vi "PH_Beckhoff_PP_PU.get Igni Tagname.vi"(1 "Igni Tag":T2, 2 "PU":T1) -> (0 "Igni Tagname":string)   [LabVIEW 2014, in "PH_Beckhoff_PP_PU.lvlib"]
doc: "This VI concatenates a Tagname out of strict type def enum controls. It keeps also the information whether the Tag is existing (if not, N/A is given out as name)."
uses:
  PH_Beckhoff_PP_PU.lvlib
  PH_Beckhoff_PP_PU.Igni Tags.ctl
  PH_PP_Common/PH_PP_Common.PUs.ctl
  PH_PP_Common/PH_PP_Common.Devices.ctl
  PH_Common/Names/PH_Names.Subsystems.ctl
  PH_Common/Names/PH_Names.Communication Type.ctl
  PH_Common/PH_Common.lvlib
  PH_PP_Common/PH_PP_Common.lvlib
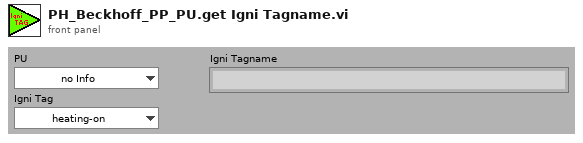
[diagram p1: front panel]
types:
  T1 = typedef "PH_PP_Common.lvlib/PH_PP_Common.PUs.ctl" = enum16{"no Info", "PA-19mm-1", "PA-19mm-2", "PA-45mm-PILC", "PA-45mm-MAIN", "MA-PU-1", "MA-PU-2", "MA-PU-3", "MA-PU-4", "MA-PU-5", "MA-PU-6", "MA-FR", "MA-PILC", "PA-45mm-DP"}
  T2 = typedef "PH_Beckhoff_PP_PU.lvlib/PH_Beckhoff_PP_PU.Igni Tags.ctl" = enum16{"heating-on", "water-on", "Device-on", "Status"}
  T3 = typedef "PH_Common.lvlib/PH_Names.Subsystems.ctl" = enum16{"no Info", "fs-FE", "ns-FE", "PA", "MA", "MAS", "COS", "Exp-LB", "Exp-LL", "PP", "PILS"}
  T4 = typedef "PH_PP_Common.lvlib/PH_PP_Common.Devices.ctl" = enum16{"no Info", "Igni", "RR", "DumpRoss", "PSU", "Trigger", "HV-Meas", "Rods", "Chiller", "Conductivity", "Mercury"}
  T5 = typedef "PH_Common.lvlib/PH_Names.Communication Type.ctl" = enum16{"no Info", "SE", "SA", "AE", "AA", "DE", "DA", "DIM"}
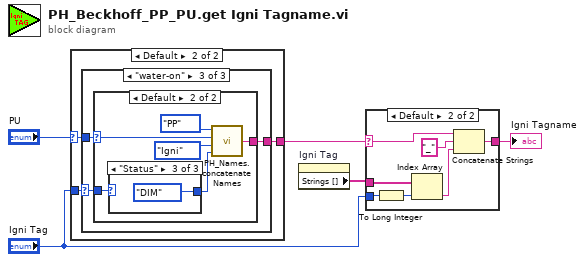
[diagram p0: block diagram]
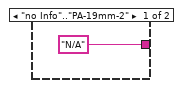
[diagram p2: hidden frame]
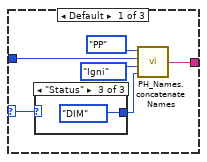
[diagram p3: hidden frame]
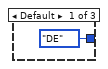
[diagram p4: hidden frame]
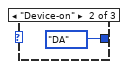
[diagram p5: hidden frame]
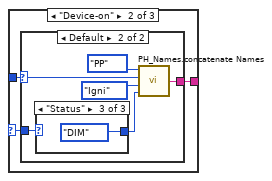
[diagram p6: hidden frame]
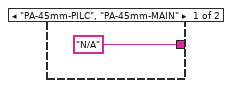
[diagram p7: hidden frame]
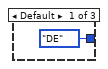
[diagram p8: hidden frame]
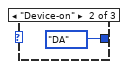
[diagram p9: hidden frame]
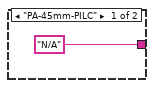
[diagram p10: hidden frame]
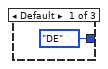
[diagram p11: hidden frame]
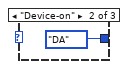
[diagram p12: hidden frame]
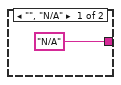
[diagram p13: hidden frame]
diagram:
  n1 = case shown="Default" "PU" {
    selector: "PU" -> [_ w8]
    tunnel: ["N/A" ("Subsystem_PU_Devices_Comm Type") w9] -> w4
    tunnel: "Igni Tag" -> [_ w7]
    frame "no Info".."PA-19mm-2" {
    }
    frame Default {
      n2 = case shown="\"water-on\"" w7 {
        selector: w7 -> [w10 w20 w33]
        tunnel: [w15 w21 w34] -> w9
        tunnel: w8 -> [w14 w19 w32]
        frame Default {
          n3 = case shown="\"Status\"" w10 {
            tunnel: [PH_Names.Communication_Type."DE" ("Communication Type (no info)") PH_Names.Communication_Type."DA" ("Communication Type (no info)") PH_Names.Communication_Type."DIM" ("Communication Type (no info)")] -> w11
            frame Default {
            }
            frame "Device-on" {
            }
            frame "Status" {
            }
          }
          n4 = call "PH_Names.concatenate Names.vi"("Communication Type (no info)"=w11, "Devices (no info)"=PH_PP_Common.Devices."Igni", "PU (no info)"=w14, "Subsystem"=PH_Names.Subsystems."PP") -> ("Subsystem_PU_Devices_Comm Type"=w15:string)
        }
        frame "Device-on" {
          n5 = case shown="Default" w19 {
            selector: w19 -> [_ w23]
            tunnel: ["N/A" ("Subsystem_PU_Devices_Comm Type") w28] -> w21
            tunnel: w20 -> [_ w24]
            frame "PA-45mm-PILC", "PA-45mm-MAIN" {
            }
            frame Default {
              n6 = case shown="\"Status\"" w24 {
                tunnel: [PH_Names.Communication_Type."DE" ("Communication Type (no info)") PH_Names.Communication_Type."DA" ("Communication Type (no info)") PH_Names.Communication_Type."DIM" ("Communication Type (no info)")] -> w25
                frame Default {
                }
                frame "Device-on" {
                }
                frame "Status" {
                }
              }
              n7 = call "PH_Names.concatenate Names.vi"("Communication Type (no info)"=w25, "Devices (no info)"=PH_PP_Common.Devices."Igni", "PU (no info)"=w23, "Subsystem"=PH_Names.Subsystems."PP") -> ("Subsystem_PU_Devices_Comm Type"=w28:string)
            }
          }
        }
        frame "water-on" {
          n8 = case shown="Default" w32 {
            selector: w32 -> [_ w36]
            tunnel: ["N/A" ("Subsystem_PU_Devices_Comm Type") w41] -> w34
            tunnel: w33 -> [_ w37]
            frame "PA-45mm-PILC" {
            }
            frame Default {
              n9 = case shown="\"Status\"" w37 {
                tunnel: [PH_Names.Communication_Type."DE" ("Communication Type (no info)") PH_Names.Communication_Type."DA" ("Communication Type (no info)") PH_Names.Communication_Type."DIM" ("Communication Type (no info)")] -> w38
                frame Default {
                }
                frame "Device-on" {
                }
                frame "Status" {
                }
              }
              n10 = call "PH_Names.concatenate Names.vi"("Communication Type (no info)"=w38, "Devices (no info)"=PH_PP_Common.Devices."Igni", "PU (no info)"=w36, "Subsystem"=PH_Names.Subsystems."PP") -> ("Subsystem_PU_Devices_Comm Type"=w41:string)
            }
          }
        }
      }
    }
  }
  n11 = property on="Igni Tag" class="Enum (strict)"() -> ("Strings []"=w3:string[])  [unwired: 2 in, 2 out]
  n12 = case shown="Default" w4 {
    selector: w4 -> [_ w46]
    tunnel: ["N/A" w52] -> w5
    tunnel: w3 -> [_ w51]
    tunnel: "Igni Tag" -> [_ w47]
    frame "", "N/A" {
    }
    frame Default {
      n13 = To Long Integer(number=w47) -> (32bit integer=w50:i32)
      n14 = Index Array(array=w51, index=w50) -> (element=w49:string)
      n15 = Concatenate Strings(w46, "_" ("string"), w49) -> (w52:string)
    }
  }
  "Igni Tagname" <- w5
